vi "Create.vi"(0 "Serialized.Text":string, 7 "Serialized.Color":u32, 11 "Serialized.Location":cluster{"x":i16, "y":i16}) -> (4 "FSM.Label":refnum<class "FSM.Label.lvclass">)   [LabVIEW 2020, in "FSM.Label.lvclass"]
uses:
  FSM.Label.lvclass
  FSM.Label.lvclass/FSM.Label.ctl
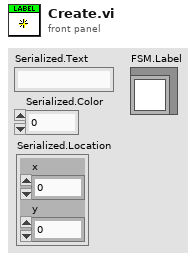
[diagram p1: front panel]
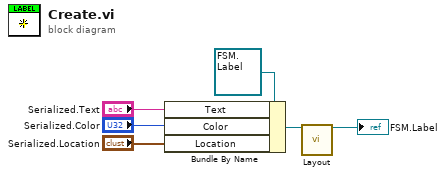
[diagram p0: block diagram]
diagram:
  n1 = Bundle By Name(cluster=refnum<class "FSM.Label.lvclass"> refnum ("FSM.Label"), "Text"="Serialized.Text", "Color"="Serialized.Color", "Location"="Serialized.Location") -> (w2:refnum<class "FSM.Label.lvclass">)
  n2 = call "Layout.vi"("FSM.Label In"=w2) -> ("FSM.Label Out"=→"FSM.Label":refnum<class "FSM.Label.lvclass">)  [unwired: 14 in]
